vi "Act.vi"(0 "Enum":enum16{"Running", "Impact", "Spinning", "Clear"}(ring)) -> ()   [LabVIEW 2010]
uses:
  UART/UART Port Type.ctl
  Main Global.vi
panel:
  out "UART port out":T1
  in  "UART port in":T1
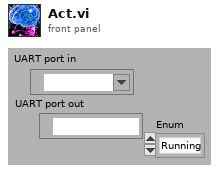
[diagram p1: front panel]
types:
  T1 = typedef "UART Port Type.ctl" = refnum<visa-resource-name>
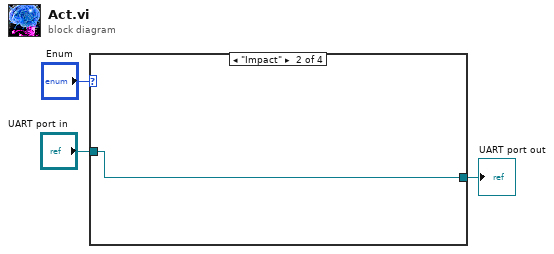
[diagram p0: block diagram]
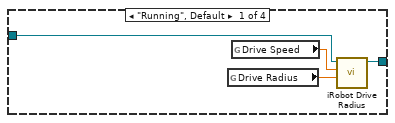
[diagram p2: hidden frame]
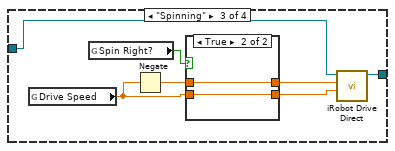
[diagram p3: hidden frame]
diagram:
  n1 = case shown="\"Impact\"" "Enum" {
    tunnel: "UART port in" -> [w7 w8 w15 w20]
    tunnel: [w6 w8 w14 w20] -> w1
    frame "Running", Default {
      n2 = global read "Main Global.vi" "Drive Radius"() -> (w5:dbl)
      n3 = global read "Main Global.vi" "Drive Speed"() -> (w4:dbl)
      n4 = call "iRobot Drive Radius.vi"("Radius (mm)"=w5, "Velocity (mm/s)"=w4, "UART port in"=w7) -> ("UART port out"=w6:T1)  [unwired: 7 in, 1 out]
    }
    frame "Impact" {
    }
    frame "Spinning" {
      n5 = global read "Main Global.vi" "Drive Speed"() -> (w9:dbl)
      n6 = global read "Main Global.vi" "Spin Right?"() -> (w12:bool)
      n7 = Negate(x=w9) -> (-x=w13:dbl)
      n8 = case shown="True" w12 {
        tunnel: [w16 w19] -> w11
        tunnel: w13 -> [w17 w19]
        tunnel: [w17 w18] -> w10
        tunnel: w9 -> [w16 w18]
        frame False {
        }
        frame True {
        }
      }
      n9 = call "iRobot Drive Direct.vi"("Left Wheel Velocity (mm/s)"=w10, "Right Wheel Velocity (mm/s)"=w11, "UART port in"=w15) -> ("UART port out"=w14:T1)  [unwired: 7 in, 1 out]
    }
    frame "Clear" {
    }
  }
  "UART port out" <- w1
